vi "PH_OceanOpticsSpectrometer.save Data to Harddisk.vi"(1 "Instance name":string, 2 "Recording Date":string, 3 "Recording Time":string, 4 "Data":dbl[][](array[numeric]), 5 "error in":errorcluster) -> (19 "error out":errorcluster)   [LabVIEW 2014, in "PH_OceanOpticsSpectrometer.lvlib"]
uses:
  PH_OceanOpticsSpectrometer.lvlib
  PH_Basics/PH_Common/Names/PH_Names.File Types.ctl
  PH_Basics/PH_Common/PH_Common.lvlib
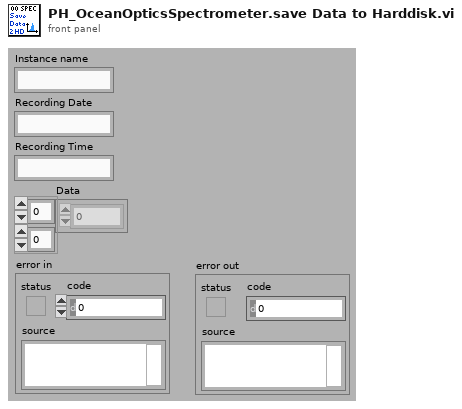
[diagram p1: front panel]
types:
  T1 = typedef "PH_Common.lvlib/PH_Names.File Types.ctl" = string
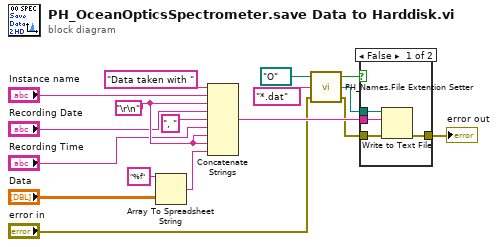
[diagram p0: block diagram]
diagram:
  w13 = "\r\n"
  n1 = Array To Spreadsheet String(array="Data", 3:"%f" ("format string")) -> (spreadsheet string=w14:string)  [unwired: 1 in]
  n2 = Concatenate Strings("Data taken with " ("string"), "Instance name", w13, "Recording Date", ", ", "Recording Time", w13, w13, w14) -> (w9:string)
  n3 = call "PH_Names.File Extention Setter.vi"("error in (no error)"="error in", "File Type"=T1 "*.dat" ("file name extinction"), "start path (O:\\)"=path "O:/" ("start path (O:\\)")) -> ("error out"=w1:errorcluster, "path with extension"=w15:path, "cancelled?"=w3:bool)
  n4 = case shown="False" w3 {
    tunnel: [w21 w22] -> w17
    tunnel: w1 -> [w20 w22]
    tunnel: w15 -> [w19 _]
    tunnel: w9 -> [w18 _]
    frame False {
      n5 = Write to Text File(file (use dialog)=w19, text=w18, error in=w20) -> (error out=w21:errorcluster)  [unwired: 1 in, 2 out]
    }
    frame True {
    }
  }
  "error out" <- w17
